vi "TEC-Temp.vi"(8 "error in (no error)":errorcluster, 11 "Stop":bool=TRUE) -> (0 "error out":errorcluster, 3 "TEC Temp [°C]":dbl)   [LabVIEW 2018]
uses:
  <vilib>/myRIO/Common/Instrument Driver Framework/myRIO v1.0/SPI/typedefs/SPI Frame Length.ctl
  <vilib>/myRIO/Common/Instrument Driver Framework/myRIO v1.0/SPI/typedefs/SPI Data Direction.ctl
  <vilib>/myRIO/Common/Instrument Driver Framework/myRIO v1.0/SPI/typedefs/SPI Clock Polarity.ctl
  <vilib>/myRIO/Common/Instrument Driver Framework/myRIO v1.0/SPI/typedefs/SPI Clock Phase.ctl
  <vilib>/myRIO/Instrument Drivers/Onboard IO/SPI/typedefs/SPI User Configuration.ctl
  <vilib>/myRIO/Instrument Drivers/Onboard IO/SPI/SPI.lvlib
  <vilib>/myRIO/Instrument Drivers/Onboard IO/SPI/typedefs/SPI Configuration.ctl
  <vilib>/myRIO/Common/Instrument Driver Framework/myRIO v1.0/SPI/typedefs/SPI Channels Enum.ctl
  <vilib>/myRIO/Common/Instrument Driver Framework/Utilities/typedefs/Generic FPGA Reference.ctl
  <vilib>/myRIO/Common/Instrument Driver Framework/Utilities/typedefs/myRIO v1.0 Reference.ctl
  <vilib>/myRIO/Common/Instrument Driver Framework/Utilities/typedefs/Hardware Version Enum.ctl
  <vilib>/myRIO/Common/Instrument Driver Framework/Utilities/typedefs/myRIO Generic Hardware Reference.ctl
  <vilib>/myRIO/Instrument Drivers/Onboard IO/SPI/typedefs/SPI Reference.ctl
  <vilib>/myRIO/Instrument Drivers/Onboard IO/SPI/vis/myRIO SPI Open.xnode
  <vilib>/userdefined/High Color/nirio_resource_hc.ctl
  <vilib>/myRIO/Instrument Drivers/Onboard IO/DIO/DIO.lvlib
  <vilib>/myRIO/Common/Instrument Driver Framework/myRIO v1.0/DIO/typedefs/DIO Channels Enum.ctl
  <vilib>/myRIO/Common/Instrument Driver Framework/myRIO v1.0/DIO/typedefs/DIO Channels List.ctl
  <vilib>/myRIO/Instrument Drivers/Onboard IO/DIO/typedefs/DIO Reference.ctl
  <vilib>/myRIO/Instrument Drivers/Onboard IO/DIO/vis/myRIO DIO Open.xnode
  <vilib>/myRIO/Common/Instrument Driver Framework/myRIO v1.0/DIO/vis/myRIO v1.1 Open DIO.vi
  <vilib>/myRIO/Common/Instrument Driver Framework/myRIO v1.0/SPI/vis/myRIO v1.1 Open SPI.vi
panel:
  in  "Stop 2":bool=TRUE
  out "Frames Read":u16[](array[numeric])
  out "CJC Temp [°C]":dbl
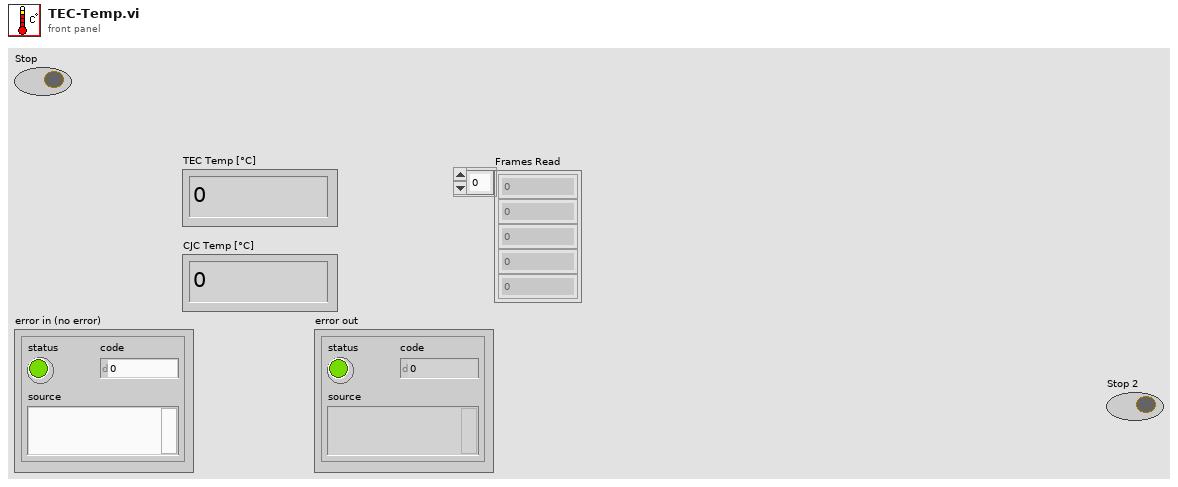
[diagram p1: front panel]
types:
  T1 = enum16{"Close Readubg", "Read", "Enable Reading", "Error Handling"}
  T2 = typedef "SPI.lvlib/SPI User Configuration.ctl" = cluster{"Frequency [Hz]":dbl, "Clock Phase":T3, "Clock Polarity":T4, "Data Direction":T5, "Frame Length":T6}
  T3 = typedef "SPI Clock Phase.ctl" = enum8{"Leading", "Trailing"}
  T4 = typedef "SPI Clock Polarity.ctl" = enum8{"Low", "High"}
  T5 = typedef "SPI Data Direction.ctl" = enum8{"Most significant bit first", "Least significant bit first"}
  T6 = typedef "SPI Frame Length.ctl" = u8
  T7 = typedef "DIO.lvlib/DIO Reference.ctl" = cluster{"myRIO Reference":T8, "DIO Channels List":T12}
  T8 = typedef "myRIO Generic Hardware Reference.ctl" = cluster{"myRIO Model":T9, "myRIO Hardware Reference":T10}
  T9 = typedef "Hardware Version Enum.ctl" = enum16{"Unknown", "myRIO-1900", "myRIO-1950", "roboRIO", "NI ELVIS RIO CM", "ELVIS III"}
  T10 = typedef "myRIO v1.0 Reference.ctl" = cluster{"Generic FPGA Reference":T11, "Allow multiple opens":bool}
  T11 = typedef "Generic FPGA Reference.ctl" = refnum<k20>
  T12 = typedef "DIO Channels List.ctl" = T13[]
  T13 = typedef "DIO Channels Enum.ctl" = enum16{"Not Connected", "C/DIO0", "C/DIO1", "C/DIO2", "C/DIO3", "C/DIO4", "C/DIO5", "C/DIO6", "C/DIO7", "A/DIO0", "A/DIO1", "A/DIO2", "A/DIO3", "A/DIO4", "A/DIO5", "A/DIO6", "A/DIO7", "A/DIO8", "A/DIO9", "A/DIO10", "A/DIO11", "A/DIO12", "A/DIO13", "A/DIO14", "A/DIO15", "A/DIO16", "A/DIO17", "A/DIO18", "A/DIO19", "B/DIO0", "B/DIO1", "B/DIO2", "B/DIO3", "B/DIO4", "B/DIO5", "B/DIO6", "B/DIO7", "B/DIO8", "B/DIO9", "B/DIO10", "B/DIO11", "B/DIO12", "B/DIO13", "B/DIO14", "B/DIO15", "B/DIO16", "B/DIO17", "B/DIO18", "B/DIO19", "LED0", "LED1", "LED2", "LED3", "Button0", "DIO/DIO0", "DIO/DIO1", "DIO/DIO2", "DIO/DIO3", "DIO/DIO4", "DIO/DIO5", "DIO/DIO6", "DIO/DIO7", "DIO/DIO8", "DIO/DIO9", "SPI/CS0", "SPI/CS1", "SPI/CS2", "SPI/CS3", "LED RADIO (Green)", "LED RADIO (Red)", "LED COMM (Green)", "LED COMM (Red)", "LED MODE (Green)", "LED MODE (Red)"}
  T14 = typedef "SPI.lvlib/SPI Reference.ctl" = cluster{"myRIO Reference":T8, "SPI Channels Enum":T15, "SPI Configuration":T16}
  T15 = typedef "SPI Channels Enum.ctl" = enum16{"Not Connected", "A/SPI", "B/SPI", "SPI/SPI"}
  T16 = typedef "SPI.lvlib/SPI Configuration.ctl" = cluster{"Frequency [Hz]":dbl, "Clock Phase":T3, "Clock Polarity":T4, "Data Direction":T5, "Frame Length":T6}
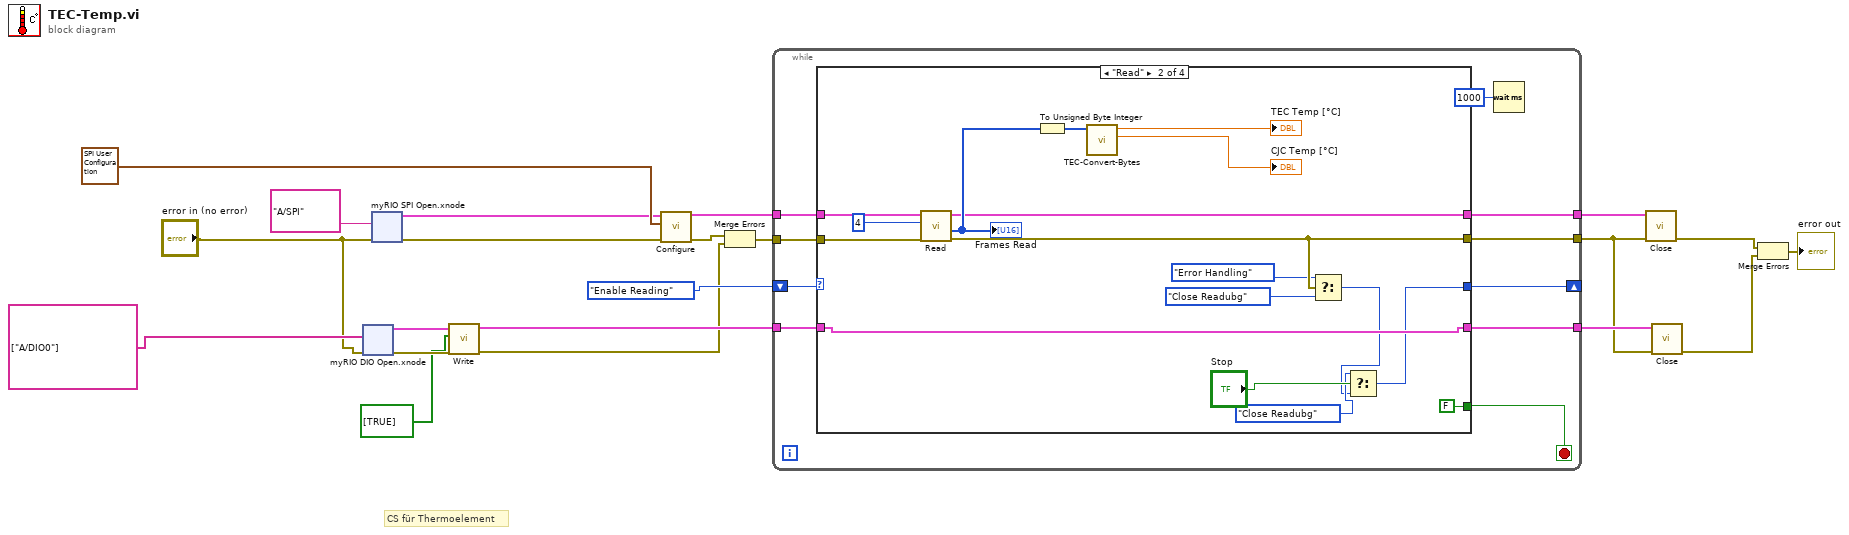
[diagram p0: block diagram]
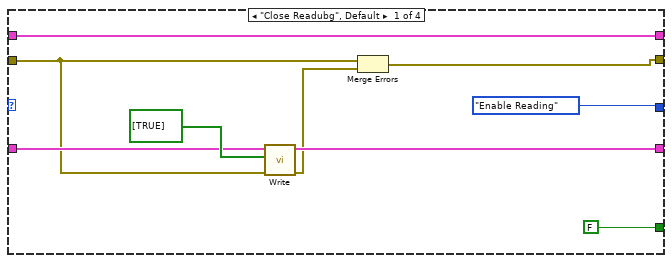
[diagram p2: hidden frame]
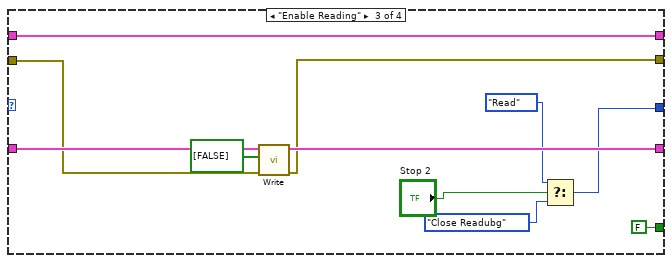
[diagram p3: hidden frame]
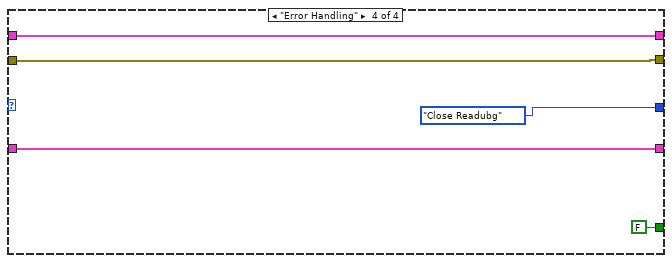
[diagram p4: hidden frame]
diagram:
  # "CS für Thermoelement"
  n1 = xnode "myRIO DIO Open.xnode"("error in (no error)"="error in (no error)", "Channel Names"=tag[] ["A/DIO0"]) -> ("error out"=w13:errorcluster, "DIO Ref Out"=w15:T7)  [unwired: 1 in]
  n2 = xnode "myRIO SPI Open.xnode"("error in (no error)"="error in (no error)", "Channel Name"=tag "A/SPI") -> ("error out"=w17:errorcluster, "SPI Ref Out"=w16:T14)  [unwired: 1 in]
  n3 = call <vilib>:"Write.vi"("error in (no error)"=w13, "Values"=bool[] [TRUE], "DIO Ref In"=w15) -> ("error out"=w7:errorcluster, "DIO Ref Out"=w9:T7)  [unwired: 6 in]
  n4 = call <vilib>:"Configure.vi"("error in (no error)"=w17, "SPI User Configuration"=T2 {"Frequency [Hz]"=1000000.0, "Clock Phase"=enum."Leading", "Clock Polarity"=enum."Low", "Data Direction"=enum."Most significant bit first", "Frame Length"=8}, "SPI Ref In"=w16) -> ("error out"=w6:errorcluster, "SPI Ref Out"=w20:T14)  [unwired: 7 in]
  n5 = Merge Errors(w6, w7) -> (w5:errorcluster)
  n6 = while {
    tunnel: w5 -> [w31]
    tunnel: w20 -> [w30]
    tunnel: [w28] -> w19
    tunnel: [w27] -> w8
    shift-right: [w22] -> _
    shift-left: T1."Enable Reading" -> [w26]
    tunnel: [w25] -> w10
    tunnel: w9 -> [w24]
    stop <- w23 stop-if-true
    n7 = case shown="\"Read\"" w26 {
      tunnel: w31 -> [w36 w55 w65 w72]
      tunnel: w30 -> [w33 w54 w63 w73]
      tunnel: [w33 w50 w63 w73] -> w28
      tunnel: [w35 w47 w64 w72] -> w27
      tunnel: [w40 w49 w68 w70] -> w25
      tunnel: w24 -> [w38 w49 w67 w70]
      tunnel: [FALSE ("Boolean") FALSE ("Boolean") FALSE ("Boolean") FALSE ("Boolean")] -> w23
      tunnel: [T1."Enable Reading" w43 w59 T1."Close Readubg"] -> w22
      frame "Close Readubg", Default {
        n8 = call <vilib>:"Write.vi"("error in (no error)"=w36, "Values"=bool[] [TRUE], "DIO Ref In"=w38) -> ("error out"=w37:errorcluster, "DIO Ref Out"=w40:T7)  [unwired: 6 in]
        n9 = Merge Errors(w36, w37) -> (w35:errorcluster)
      }
      frame "Read" {
        n10 = call <vilib>:"Read.vi"("error in (no error)"=w55, "Frame Count"=u32 4, "SPI Ref In"=w54) -> ("error out"=w47:errorcluster, "Frames Read"=w52:u16[], "SPI Ref Out"=w50:T14)  [unwired: 5 in]
        "Frames Read" <- w52
        n11 = To Unsigned Byte Integer(number=w52) -> (unsigned 8bit integer=w53:u8[])
        n12 = call "TEC-Convert-Bytes.vi"("Frames Read"=w53) -> ("CJC Temp [°C]"=→"CJC Temp [°C]":dbl, "TEC Temp [°C]"=→"TEC Temp [°C]":dbl)  [unwired: 5 in, 4 out]
        n13 = Select(t=T1."Error Handling", s=w47, f=T1."Close Readubg") -> (s? t:f=w41:T1)
        n14 = Select(t=T1."Close Readubg", s="Stop", f=w41) -> (s? t:f=w43:T1)
      }
      frame "Enable Reading" {
        n15 = call <vilib>:"Write.vi"("error in (no error)"=w65, "Values"=bool[] [FALSE], "DIO Ref In"=w67) -> ("error out"=w64:errorcluster, "DIO Ref Out"=w68:T7)  [unwired: 6 in]
        n16 = Select(t=T1."Read", s="Stop 2", f=T1."Close Readubg") -> (s? t:f=w59:T1)
      }
      frame "Error Handling" {
      }
    }
    n17 = Wait (ms)(milliseconds to wait=u32 1000) -> ()  [unwired: 1 out]
  }
  n18 = call <vilib>:"Close.vi"("error in (no error)"=w8, "SPI Ref In"=w19) -> ("error out"=w3:errorcluster)  [unwired: 9 in]
  n19 = call <vilib>:"Close.vi"("error in (no error)"=w8, "DIO Ref In"=w10) -> ("error out"=w2:errorcluster)  [unwired: 9 in]
  n20 = Merge Errors(w3, w2) -> (→"error out":errorcluster)
